vi "add points int.vi"(5 "Overwrite Lib Path":path, 6 "rebuild_threshold":sgl=1.0, 8 "error in (no error)":errorcluster, 10 "points":i32[][](array[numeric]), 11 "index_ptr":u64) -> (0 "error out":errorcluster, 3 "index_ptr out":u64)   [LabVIEW 2020, in "KD Tree.lvlib"]
doc: "FLANN_EXPORT int flann_add_points_double(flann_index_t index_ptr,\n double* points, int rows, int columns,\n float rebuild_threshold);"
uses:
  KD Tree.lvlib
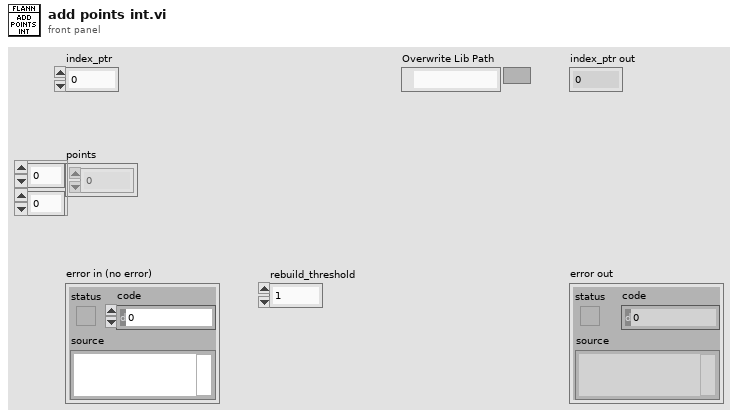
[diagram p1: front panel]
types:
  T1 = typedef "Semaphore RefNum" = refnum<k1>
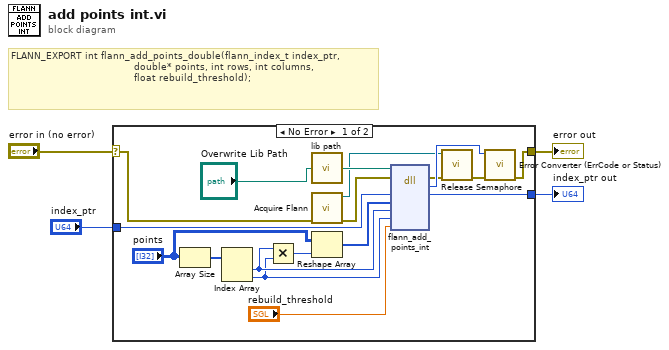
[diagram p0: block diagram]
diagram:
  # "FLANN_EXPORT int flann_add_points_double(flann_index_t index_ptr,\n                                         double* points, int rows, int columns,\n                                         float rebuild_threshold);"
  n1 = case shown="No Error" "error in (no error)" {
    selector: "error in (no error)" -> [w21 w24]
    tunnel: [w19 w24] -> w3
    tunnel: [w18 w23] -> w2
    tunnel: "index_ptr" -> [w10 w23]
    frame No Error {
      n2 = Array Size(array="points") -> (size(s)=w16:i32[])
      n3 = Index Array(array=w16) -> (element #1=w14:i32, element #2=w13:i32)  [unwired: 2 in]
      n4 = Multiply(x=w14, y=w13) -> (x*y=w11:i32)
      n5 = call "lib path.vi"("Overwrite Lib Path"="Overwrite Lib Path") -> ("lib path"=w9:path)
      n6 = call "Acquire Flann.vi"("error in (no error)"=w21) -> ("error out"=w7:errorcluster, "semaphore"=w5:T1)  [unwired: 9 in]
      n7 = Reshape Array("points", w11) -> (w15:i32[])
      n8 = dll-call lib="E:/Labview/LV 2020/Libs/flann/flann.*" fn="flann_add_points_int"(path in=w9, error in=w7, "index_ptr"=w10, "points"=w15, "rows"=w14, "columns"=w13, "rebuild_threshold"="rebuild_threshold") -> (error out=w20:errorcluster, "return type"=w22:i32, "index_ptr"=w18:u64)  [unwired: 5 in, 1 out]
      n9 = call <vilib>:"Release Semaphore.vi"("error in (no error)"=w20, "semaphore"=w5) -> ("error out"=w6:errorcluster)  [unwired: 4 in, 1 out]
      n10 = call "Error Converter (ErrCode or Status).vi"("error in (no error)"=w6, "error code"=w22) -> ("error out"=w19:errorcluster)  [unwired: 9 in]
    }
    frame Error {
    }
  }
  "error out" <- w3
  "index_ptr out" <- w2
